vi "LC Excel Read.vi"(8 "error in (no error)":errorcluster caption="错误输入（无错误）", 9 "worksheet index (0)":i32, 11 "Path":path=path "E:/AgainDo/项目/进行中/莱茵化学FCM报价系统/FCM 2021.08.26/Document/材料管理文件.xlsx") -> (0 "error out":errorcluster caption="错误输出", 2 "Read":string[][](array[string]))   [LabVIEW 2020]
uses:
  <vilib>/Utility/NIReport.llb/Report Type.ctl
  <vilib>/addons/_office/excel.llb/Excel Get Data ([str]).vi
  <vilib>/Utility/NIReport.llb/NI_report.lvclass
  <vilib>/Utility/NIReport.llb/NI_ReportGenerationCore.lvlib
  <vilib>/Utility/NIReport.llb/Excel/NI_Excel.lvclass
  <vilib>/addons/_office/NI_ReportGenerationToolkit.lvlib
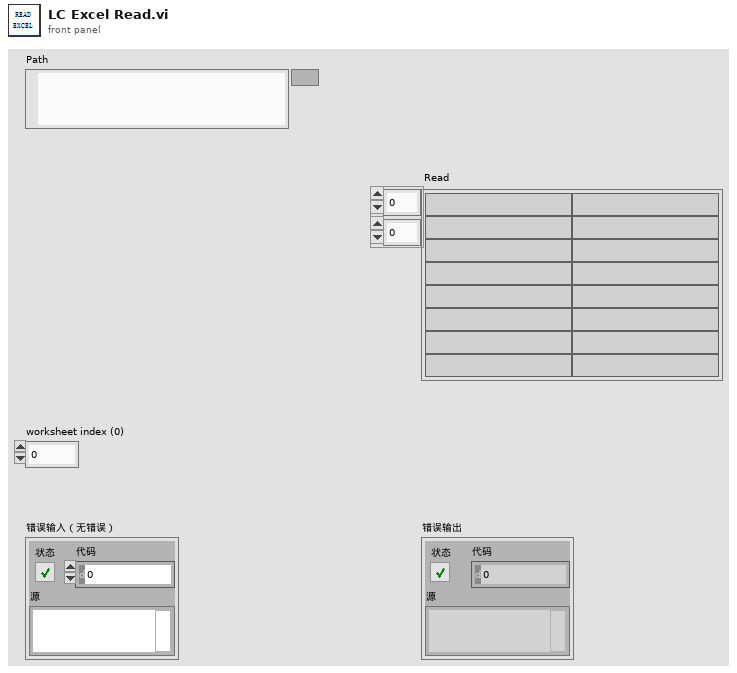
[diagram p1: front panel]
types:
  T1 = enum16{"maximized", "minimized", "normal", "no change"}
  T2 = typedef "NI_ReportGenerationCore.lvlib/Report Type.ctl" = enum16{"HTML", "Word", "Excel"}
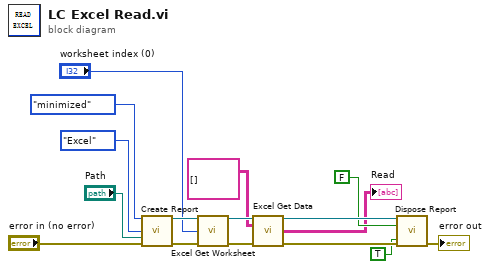
[diagram p0: block diagram]
diagram:
  n1 = call <vilib>:"Create Report.vi"("window state (normal)"=T1."minimized", "report type"=Report_Type."Excel", "template (empty)"="Path", "error in (no error)"="error in (no error)") -> ("report out"=w11:refnum<class "NI_report.lvclass">, "error out"=w10:errorcluster)  [unwired: 10 in]
  n2 = call <vilib>:"Excel Get Worksheet.vi"("report in"=w11, "worksheet index (0)"="worksheet index (0)", "error in (no error)"=w10) -> ("report out"=w6:refnum<class "NI_report.lvclass">, "error out"=w5:errorcluster)  [unwired: 11 in]
  n3 = call-poly <vilib>:"Excel Get Data.vi"("report in"=w6, "data type"=string[][] [], "error in (no error)"=w5) -> ("report out"=w9:refnum<class "NI_report.lvclass">, "data"=→"Read":string[][], "error out"=w8:errorcluster)  [unwired: 10 in]
  n4 = call-dynamic "Dispose Report.vi"("report in"=w9, "wait until printing completed? (T)"=FALSE, "error in (no error)"=w8, "close report? (T)"=TRUE) -> ("error out"=→"error out":errorcluster)  [unwired: 11 in]
